vi "SetArmHomeStatus.vi"(1 "ArmHomeFailure":bool, 2 "ArmHomeSuccess":bool) -> ()   [LabVIEW 2017]
uses:
  <vilib>/Rock Robotics/Network Tables/NT Write Boolean.vi
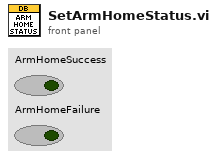
[diagram p1: front panel]
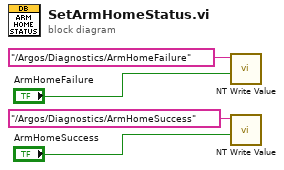
[diagram p0: block diagram]
diagram:
  n1 = call-poly <vilib>:"NT Write Value.vi"("Boolean"="ArmHomeFailure", "Name"="/Argos/Diagnostics/ArmHomeFailure") -> ()  [unwired: 9 in, 1 out]
  n2 = call-poly <vilib>:"NT Write Value.vi"("Boolean"="ArmHomeSuccess", "Name"="/Argos/Diagnostics/ArmHomeSuccess") -> ()  [unwired: 9 in, 1 out]
